vi "Update Lamp NP.vi"(8 "error in (no error)":errorcluster, 11 "Lamp Container In":refnum<class "Lamp Container.lvclass">) -> (0 "error out":errorcluster, 2 "Lamps":T1, 3 "Lamp Container Out":refnum<class "Lamp Container.lvclass">)   [LabVIEW 2016]
uses:
  Controls/All Lamps.ctl
  Controls/Lamp Data.ctl
  Classes/Lamp/Container/Lamp Container.lvclass
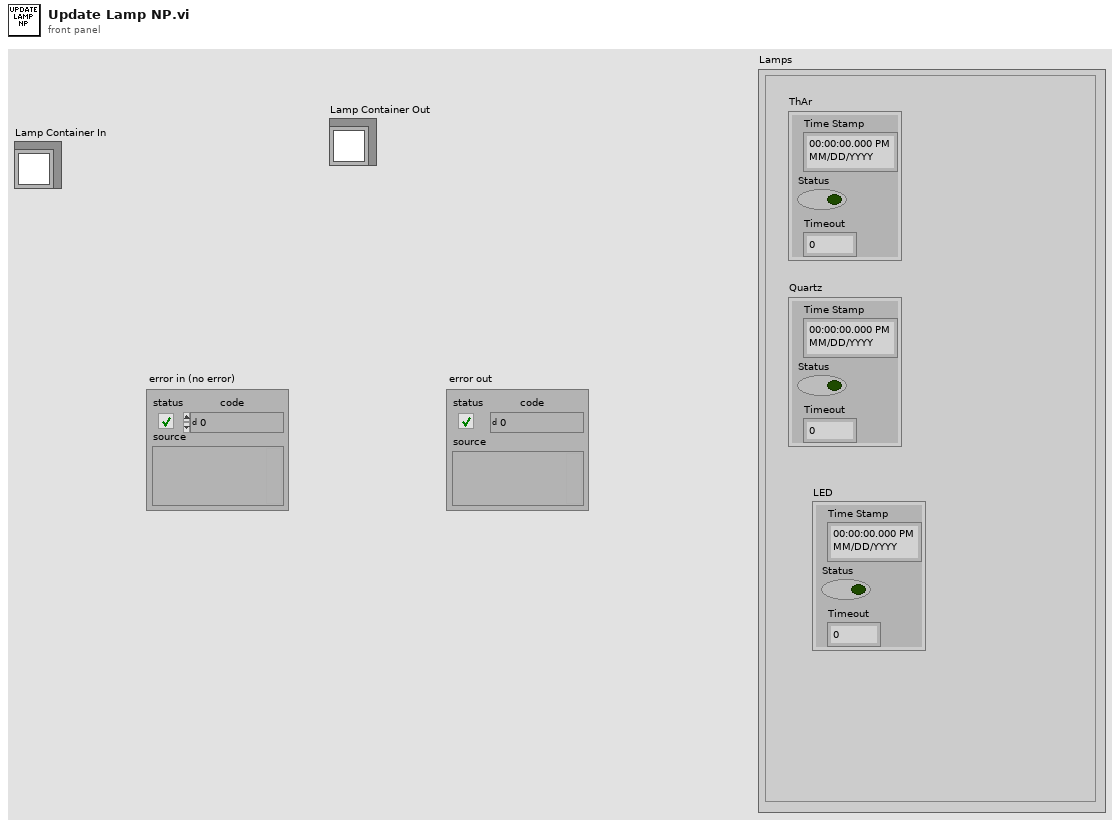
[diagram p1: front panel]
types:
  T1 = typedef "All Lamps.ctl" = cluster{"Lamp":T2, "Quartz":T2, "LED":T2}
  T2 = typedef "Lamp Data.ctl" = cluster{"Time Stamp":timestamp, "Status":bool, "Timeout":dbl}
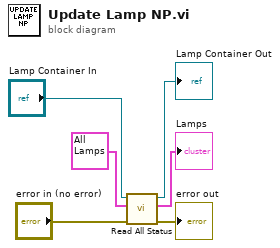
[diagram p0: block diagram]
diagram:
  n1 = call-dynamic "Read All Status.vi"("error in (no error)"="error in (no error)", "Lamps In"=T1 {"Lamp"={"Time Stamp"=timestamp(0 s since 1904-01-01), "Status"=FALSE, "Timeout"=0.0}, "Quartz"={"Time Stamp"=timestamp(0 s since 1904-01-01), "Status"=FALSE, "Timeout"=0.0}, "LED"={"Time Stamp"=timestamp(0 s since 1904-01-01), "Status"=FALSE, "Timeout"=0.0}} ("Lamps 2"), "Lamp Container in"="Lamp Container In") -> ("error out"=→"error out":errorcluster, "Lamps Out"=→"Lamps":T1, "Lamp Container out"=→"Lamp Container Out":refnum<class "Lamp Container.lvclass">)  [unwired: 6 in]
